vi "Find Label by Name.vi"(8 "error in":errorcluster, 10 "label name":string, 11 "port in":T1 format="%.0x") -> (0 "error out":errorcluster, 2 "label":T1 format="%.0x", 3 "port out":T1 format="%.0x", 4 "found?":bool)   [LabVIEW 2020, in "Ballard ARINC 429 Scripting.lvlib"]
doc: "Under the specified port, searches for a label with matching <b>label name</b>. If a match is found, the reference to the matching label is returned. If no match is found, the returned reference is invalid and <b>found?</b> equals False."
uses:
  Ballard ARINC 429 Scripting.lvlib
  <vilib>/NI VeriStand/Custom Device API/Custom Device Item Ref.ctl
  <vilib>/NI VeriStand/Custom Device Tools/Custom Device Utility Library/NI VeriStand - Search for Item by Name.vi
  <vilib>/NI VeriStand/Custom Device Tools/Custom Device Utility Library/Custom Device Utility Library.lvlib
  <vilib>/NI VeriStand/Custom Device API/Custom Device API.lvlib
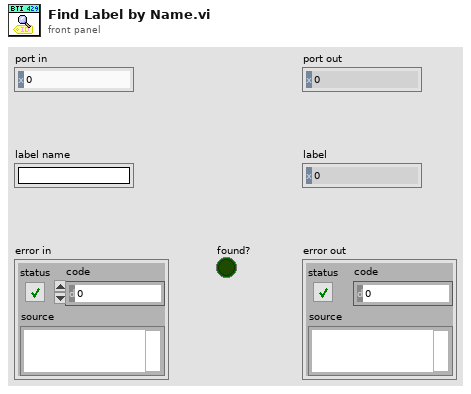
[diagram p1: front panel]
types:
  T1 = typedef "Custom Device API.lvlib/Custom Device Item Ref.ctl" = u64
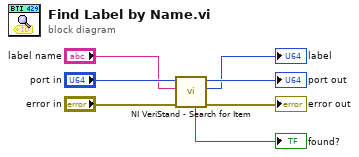
[diagram p0: block diagram]
diagram:
  n1 = call-poly <vilib>:"NI VeriStand - Search for Item.vi"("error in"="error in", "Item Name"="label name", "Section Ref in"="port in") -> ("error out"=→"error out":errorcluster, "Item Ref"=→"label":T1, "Section Ref out"=→"port out":T1, "Found"=→"found?":bool)  [unwired: 5 in]
